vi "LoadPodDriveData.vi"(9 "Pod Number":i32, 10 "Pod Configuration in":T2, 11 "Config file Refnum in":T1) -> (2 "Pod Configuration out":T2, 3 "Config file Refnum out":T1)   [LabVIEW 2014]
uses:
  <vilib>/Utility/config.llb/Config Data RefNum.ctl
  <vilib>/Utility/config.llb/Read Key (Boolean).vi
  <vilib>/Utility/config.llb/Write Key (Boolean).vi
  <vilib>/Utility/config.llb/Read Key (I32).vi
  <vilib>/Utility/config.llb/Write Key (I32).vi
  <vilib>/Utility/config.llb/Read Key (Double).vi
  <vilib>/Utility/config.llb/Write Key (Double).vi
  <vilib>/Utility/config.llb/Read Key (String).vi
  <vilib>/Utility/config.llb/Write Key (String).vi
  <vilib>/Utility/config.llb/NI_LVConfig.lvlib
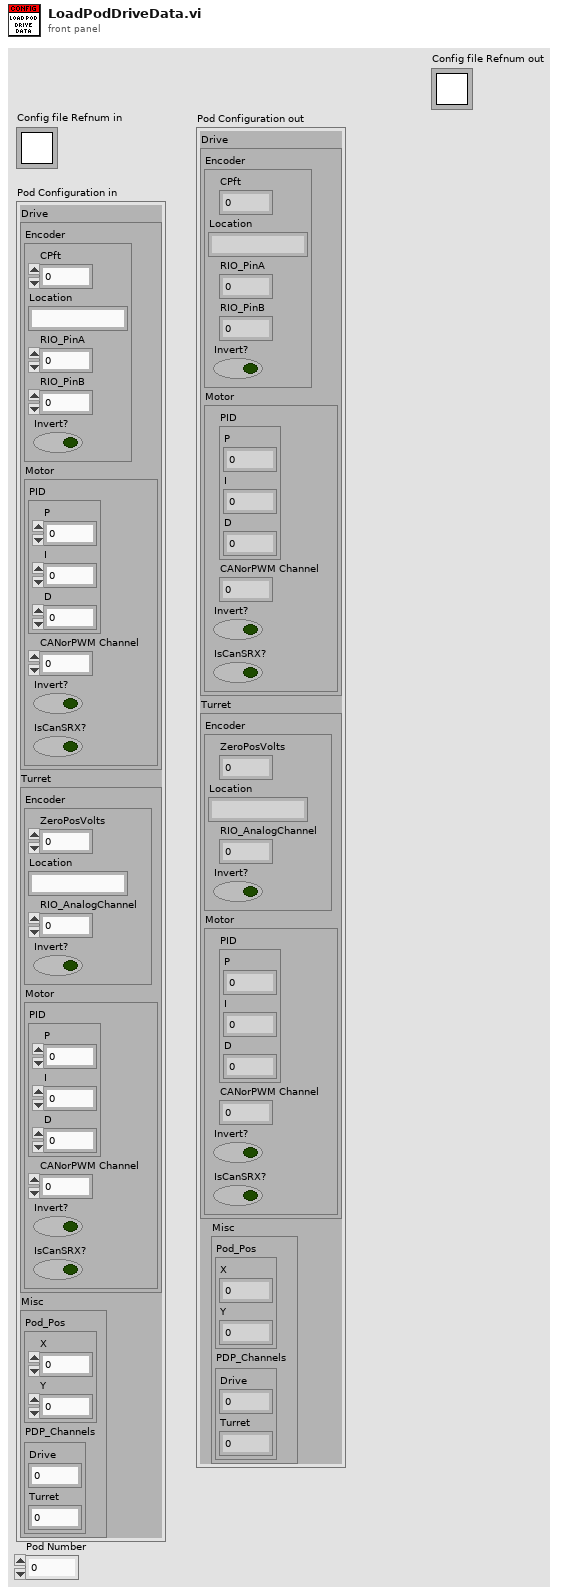
[diagram p1: front panel]
types:
  T1 = typedef "NI_LVConfig.lvlib/Config Data RefNum.ctl" = refnum<k1>
  T2 = cluster{"Drive":cluster{"Encoder":cluster{"CPft":dbl, "Location":string, "RIO_PinA":i32, "RIO_PinB":i32, "Invert?":bool}, "Motor":cluster{"PID":cluster{"P":dbl, "I":dbl, "D":dbl}, "CANorPWM Channel":i32, "Invert?":bool, "IsCanSRX?":bool}}, "Turret":cluster{"Encoder":cluster{"ZeroPosVolts":dbl, "Location":string, "RIO_AnalogChannel":i32, "Invert?":bool}, "Motor":cluster{"PID":cluster{"P":dbl, "I":dbl, "D":dbl}, "CANorPWM Channel":i32, "Invert?":bool, "IsCanSRX?":bool}}, "Misc":cluster{"Pod_Pos":cluster{"X":dbl, "Y":dbl}, "PDP_Channels":cluster{"Drive":i32, "Turret":i32}}}
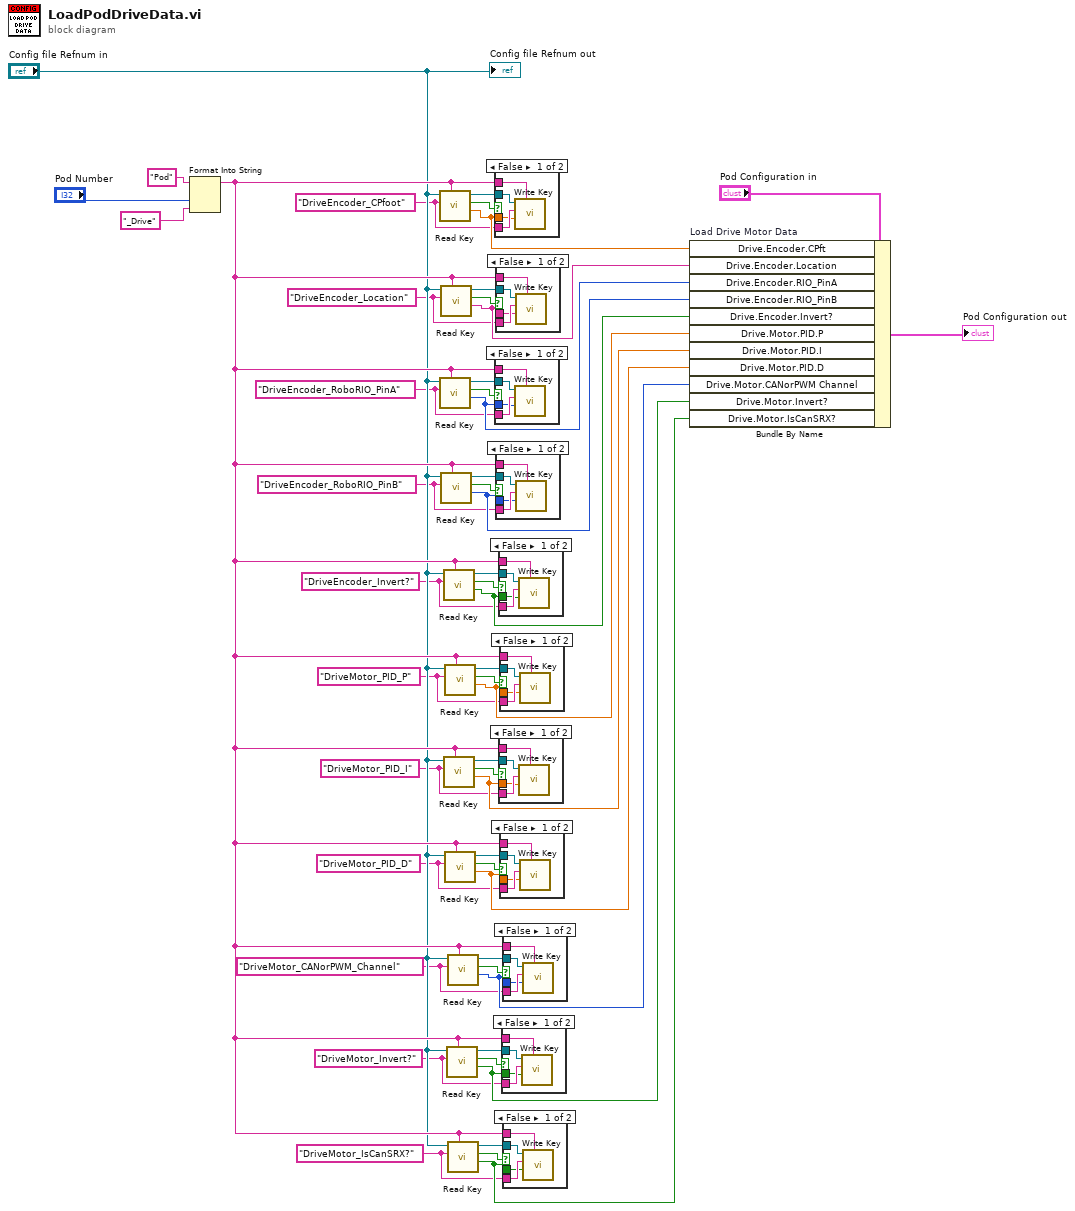
[diagram p0: block diagram]
diagram:
  w42 = "DriveMotor_IsCanSRX?" ("string")
  w43 = "DriveMotor_Invert?" ("string")
  w37 = "DriveMotor_CANorPWM_Channel" ("string")
  w24 = "DriveMotor_PID_D" ("string")
  w23 = "DriveMotor_PID_I" ("string")
  w29 = "DriveMotor_PID_P" ("string")
  w30 = "DriveEncoder_Invert?" ("string")
  w15 = "DriveEncoder_RoboRIO_PinB" ("string")
  w16 = "DriveEncoder_RoboRIO_PinA" ("string")
  w8 = "DriveEncoder_Location" ("string")
  w7 = "DriveEncoder_CPfoot" ("string")
  n1 = Format Into String(initial string="Pod", "Pod Number", "_Drive") -> (resulting string=w50:string)  [unwired: 2 in, 1 out]
  n2 = call-poly <vilib>:"Read Key.vi"("section"=w50, "key"=w7, "refnum"="Config file Refnum in") -> ("value"=w11:dbl, "found?"=w5:bool, "refnum out"=w6:T1)  [unwired: 5 in, 1 out]
  n3 = call-poly <vilib>:"Read Key.vi"("section"=w50, "key"=w16, "refnum"="Config file Refnum in") -> ("value"=w19:i32, "found?"=w18:bool, "refnum out"=w17:T1)  [unwired: 5 in, 1 out]
  n4 = call-poly <vilib>:"Read Key.vi"("section"=w50, "key"=w8, "refnum"="Config file Refnum in") -> ("value"=w12:string, "found?"=w10:bool, "refnum out"=w9:T1)  [unwired: 5 in, 1 out]
  n5 = call-poly <vilib>:"Read Key.vi"("section"=w50, "key"=w15, "refnum"="Config file Refnum in") -> ("value"=w20:i32, "found?"=w13:bool, "refnum out"=w14:T1)  [unwired: 5 in, 1 out]
  n6 = call-poly <vilib>:"Read Key.vi"("section"=w50, "key"=w30, "refnum"="Config file Refnum in") -> ("value"=w33:bool, "found?"=w32:bool, "refnum out"=w31:T1)  [unwired: 5 in, 1 out]
  n7 = call-poly <vilib>:"Read Key.vi"("section"=w50, "key"=w23, "refnum"="Config file Refnum in") -> ("value"=w35:dbl, "found?"=w21:bool, "refnum out"=w22:T1)  [unwired: 5 in, 1 out]
  n8 = call-poly <vilib>:"Read Key.vi"("section"=w50, "key"=w29, "refnum"="Config file Refnum in") -> ("value"=w34:dbl, "found?"=w27:bool, "refnum out"=w28:T1)  [unwired: 5 in, 1 out]
  n9 = call-poly <vilib>:"Read Key.vi"("section"=w50, "key"=w24, "refnum"="Config file Refnum in") -> ("value"=w36:dbl, "found?"=w26:bool, "refnum out"=w25:T1)  [unwired: 5 in, 1 out]
  n10 = call-poly <vilib>:"Read Key.vi"("section"=w50, "key"=w43, "refnum"="Config file Refnum in") -> ("value"=w48:bool, "found?"=w45:bool, "refnum out"=w44:T1)  [unwired: 5 in, 1 out]
  n11 = call-poly <vilib>:"Read Key.vi"("section"=w50, "key"=w37, "refnum"="Config file Refnum in") -> ("value"=w47:i32, "found?"=w39:bool, "refnum out"=w38:T1)  [unwired: 5 in, 1 out]
  n12 = call-poly <vilib>:"Read Key.vi"("section"=w50, "key"=w42, "refnum"="Config file Refnum in") -> ("value"=w49:bool, "found?"=w40:bool, "refnum out"=w41:T1)  [unwired: 5 in, 1 out]
  n13 = case shown="False" w5 {
    tunnel: w6 -> [w55 _]
    tunnel: w50 -> [w54 _]
    tunnel: w7 -> [w53 _]
    tunnel: w11 -> [w52 _]
    frame False {
      n14 = call-poly <vilib>:"Write Key.vi"("section"=w54, "value"=w52, "key"=w53, "refnum"=w55) -> ()  [unwired: 5 in, 3 out]
    }
    frame True {
    }
  }
  n15 = case shown="False" w18 {
    tunnel: w17 -> [w59 _]
    tunnel: w50 -> [w58 _]
    tunnel: w16 -> [w57 _]
    tunnel: w19 -> [w56 _]
    frame False {
      n16 = call-poly <vilib>:"Write Key.vi"("section"=w58, "value"=w56, "key"=w57, "refnum"=w59) -> ()  [unwired: 5 in, 3 out]
    }
    frame True {
    }
  }
  n17 = case shown="False" w10 {
    tunnel: w9 -> [w63 _]
    tunnel: w50 -> [w62 _]
    tunnel: w8 -> [w61 _]
    tunnel: w12 -> [w60 _]
    frame False {
      n18 = call-poly <vilib>:"Write Key.vi"("section"=w62, "value"=w60, "key"=w61, "refnum"=w63) -> ()  [unwired: 5 in, 3 out]
    }
    frame True {
    }
  }
  n19 = case shown="False" w13 {
    tunnel: w14 -> [w67 _]
    tunnel: w50 -> [w66 _]
    tunnel: w15 -> [w65 _]
    tunnel: w20 -> [w64 _]
    frame False {
      n20 = call-poly <vilib>:"Write Key.vi"("section"=w66, "value"=w64, "key"=w65, "refnum"=w67) -> ()  [unwired: 5 in, 3 out]
    }
    frame True {
    }
  }
  n21 = case shown="False" w32 {
    tunnel: w31 -> [w71 _]
    tunnel: w50 -> [w70 _]
    tunnel: w30 -> [w69 _]
    tunnel: w33 -> [w68 _]
    frame False {
      n22 = call-poly <vilib>:"Write Key.vi"("section"=w70, "value"=w68, "key"=w69, "refnum"=w71) -> ()  [unwired: 5 in, 3 out]
    }
    frame True {
    }
  }
  n23 = case shown="False" w21 {
    tunnel: w22 -> [w75 _]
    tunnel: w50 -> [w74 _]
    tunnel: w23 -> [w73 _]
    tunnel: w35 -> [w72 _]
    frame False {
      n24 = call-poly <vilib>:"Write Key.vi"("section"=w74, "value"=w72, "key"=w73, "refnum"=w75) -> ()  [unwired: 5 in, 3 out]
    }
    frame True {
    }
  }
  n25 = case shown="False" w27 {
    tunnel: w28 -> [w79 _]
    tunnel: w50 -> [w78 _]
    tunnel: w29 -> [w77 _]
    tunnel: w34 -> [w76 _]
    frame False {
      n26 = call-poly <vilib>:"Write Key.vi"("section"=w78, "value"=w76, "key"=w77, "refnum"=w79) -> ()  [unwired: 5 in, 3 out]
    }
    frame True {
    }
  }
  n27 = case shown="False" w26 {
    tunnel: w25 -> [w83 _]
    tunnel: w50 -> [w82 _]
    tunnel: w24 -> [w81 _]
    tunnel: w36 -> [w80 _]
    frame False {
      n28 = call-poly <vilib>:"Write Key.vi"("section"=w82, "value"=w80, "key"=w81, "refnum"=w83) -> ()  [unwired: 5 in, 3 out]
    }
    frame True {
    }
  }
  n29 = case shown="False" w45 {
    tunnel: w44 -> [w87 _]
    tunnel: w50 -> [w86 _]
    tunnel: w43 -> [w85 _]
    tunnel: w48 -> [w84 _]
    frame False {
      n30 = call-poly <vilib>:"Write Key.vi"("section"=w86, "value"=w84, "key"=w85, "refnum"=w87) -> ()  [unwired: 5 in, 3 out]
    }
    frame True {
    }
  }
  n31 = case shown="False" w39 {
    tunnel: w38 -> [w91 _]
    tunnel: w50 -> [w90 _]
    tunnel: w37 -> [w89 _]
    tunnel: w47 -> [w88 _]
    frame False {
      n32 = call-poly <vilib>:"Write Key.vi"("section"=w90, "value"=w88, "key"=w89, "refnum"=w91) -> ()  [unwired: 5 in, 3 out]
    }
    frame True {
    }
  }
  n33 = case shown="False" w40 {
    tunnel: w41 -> [w95 _]
    tunnel: w50 -> [w94 _]
    tunnel: w42 -> [w93 _]
    tunnel: w49 -> [w92 _]
    frame False {
      n34 = call-poly <vilib>:"Write Key.vi"("section"=w94, "value"=w92, "key"=w93, "refnum"=w95) -> ()  [unwired: 5 in, 3 out]
    }
    frame True {
    }
  }
  n35 = Bundle By Name "Load Drive Motor Data"(cluster="Pod Configuration in", "Drive.Encoder.CPft"=w11, "Drive.Encoder.Location"=w12, "Drive.Encoder.RIO_PinA"=w19, "Drive.Encoder.RIO_PinB"=w20, "Drive.Encoder.Invert?"=w33, "Drive.Motor.PID.P"=w34, "Drive.Motor.PID.I"=w35, "Drive.Motor.PID.D"=w36, "Drive.Motor.CANorPWM Channel"=w47, "Drive.Motor.Invert?"=w48, "Drive.Motor.IsCanSRX?"=w49) -> (→"Pod Configuration out":T2)
  "Config file Refnum out" <- "Config file Refnum in"
